vi "TimeStampToString.vi"(7 "形式":enum16{"年～秒", "時:～.ミリ秒"}(ring), 11 "タイムスタンプ":timestamp) -> (3 "日付/時間文字列":string)   [LabVIEW 2014]
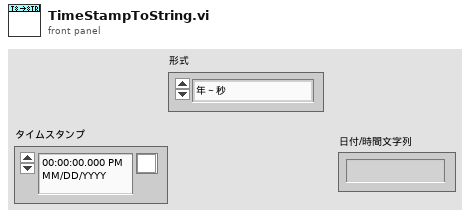
[diagram p1: front panel]
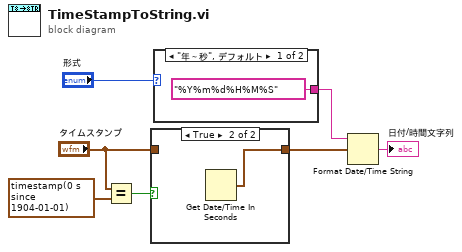
[diagram p0: block diagram]
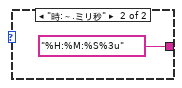
[diagram p3: hidden frame]
diagram:
  n1 = Equal?(x="タイムスタンプ", y=timestamp(0 s since 1904-01-01)) -> (x = y?=w3:bool)
  n2 = case shown="TRUE" w3 {
    tunnel: "タイムスタンプ" -> [w8 _]
    tunnel: [w8 w9] -> w1
    frame False {
    }
    frame True {
      n3 = Get Date/Time In Seconds() -> (seconds since 1Jan1904=w9:timestamp)
    }
  }
  n4 = case shown="\"年～秒\", デフォルト" "形式" {
    tunnel: ["%Y%m%d%H%M%S" ("時間形式文字列（%c）") "%H:%M:%S%3u" ("時間形式文字列（%c）")] -> w7
    frame "年～秒", Default {
    }
    frame "時:～.ミリ秒" {
    }
  }
  n5 = Format Date/Time String(time format string (%c)=w7, seconds (now)=w1) -> (date/time string=→"日付/時間文字列":string)  [unwired: 1 in]
